vi "Inventario.vi"(8 "error in (no error)":errorcluster, 10 "Numeric":u16, 11 "LHL Actor in":refnum<class "LHL Actor.lvclass">) -> (0 "error out":errorcluster, 3 "LHL Actor out":refnum<class "LHL Actor.lvclass">)   [LabVIEW 2020, in "LHL Actor.lvlib" / "LHL Actor.lvclass"]
uses:
  LHL Actor.lvclass
  LHL Actor.lvclass/LHL Actor.ctl
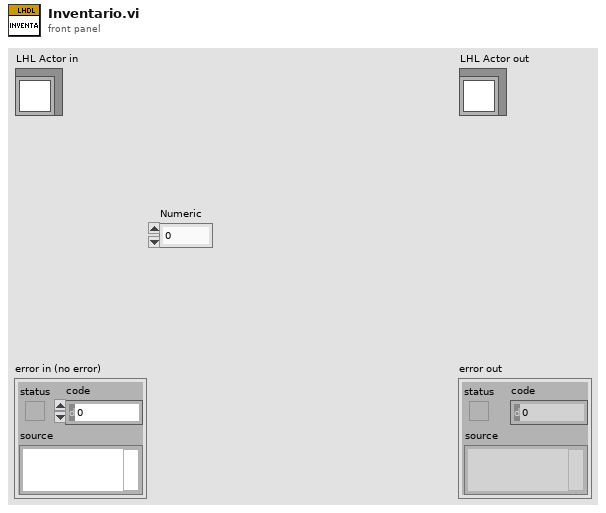
[diagram p1: front panel]
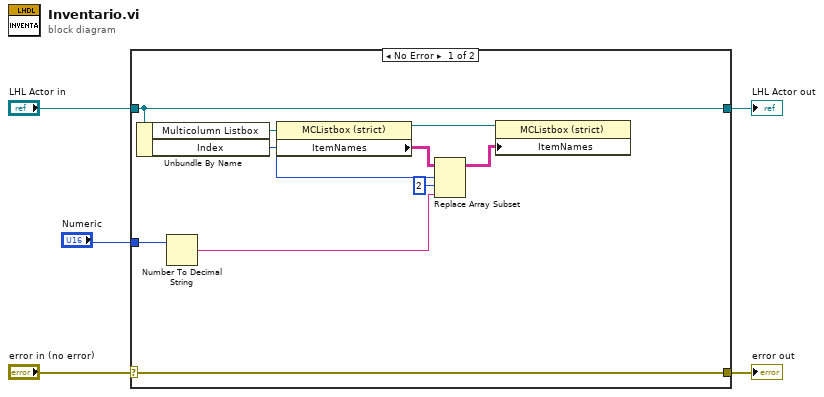
[diagram p0: block diagram]
diagram:
  n1 = case shown="No Error" "error in (no error)" {
    selector: "error in (no error)" -> [w15 w17]
    tunnel: [w15 w17] -> w4
    tunnel: [w14 w16] -> w2
    tunnel: "LHL Actor in" -> [w14 w16]
    tunnel: "Numeric" -> [w9 _]
    frame No Error {
      n2 = Unbundle By Name(w14) -> ("Multicolumn Listbox"=w13:refnum<vi>, "Index"=w11:u16)
      n3 = Number To Decimal String(number=w9) -> (decimal integer string=w8:string)  [unwired: 1 in]
      n4 = property class="MCListbox (strict)"(reference=w13) -> (reference out=w6:refnum<vi>, "ItemNames"=w12:string[][])  [unwired: 1 in, 1 out]
      n5 = Replace Array Subset(array=w12, new element=w8, index (row)=w11, index (col)=2 ("disabled index (col)")) -> (w7:string[][])
      n6 = property class="MCListbox (strict)"(reference=w6, "ItemNames"=w7) -> ()  [unwired: 1 in, 2 out]
    }
    frame Error {
    }
  }
  "error out" <- w4
  "LHL Actor out" <- w2
